vi "Host_17 - Copy - Copy.vi"() -> ()   [LabVIEW 2017]
uses:
  <vilib>/Platform/browser.llb/Open URL in Default Browser (string).vi
  <vilib>/lvdsc/tagapi/classes/Tag Reader/Tag Reader.lvclass
panel:
  in  "stop":bool
  out "Motor Speed":cluster{i32, dbl}[](graph)
  out "Armature Current":cluster{i32, dbl}[](graph)
  out "Feedback Load Torque 2":dbl
  out "Feedback Duty Cycle 2":dbl
  in  "Duty Cycle 2":dbl(slide) scale=0.0..100.0
  in  "Load Torque 2":dbl(slide) scale=-0.2..0.2
  in  "Data Update Speed (ms)":dbl
  in  "Website Button":bool
  in  "Doc Button":bool
  in  "Save Button":bool
  in  "Run Button":bool
  # "OPAL-RT Real Time Outputs"
  # "Microcontroller Inputs"
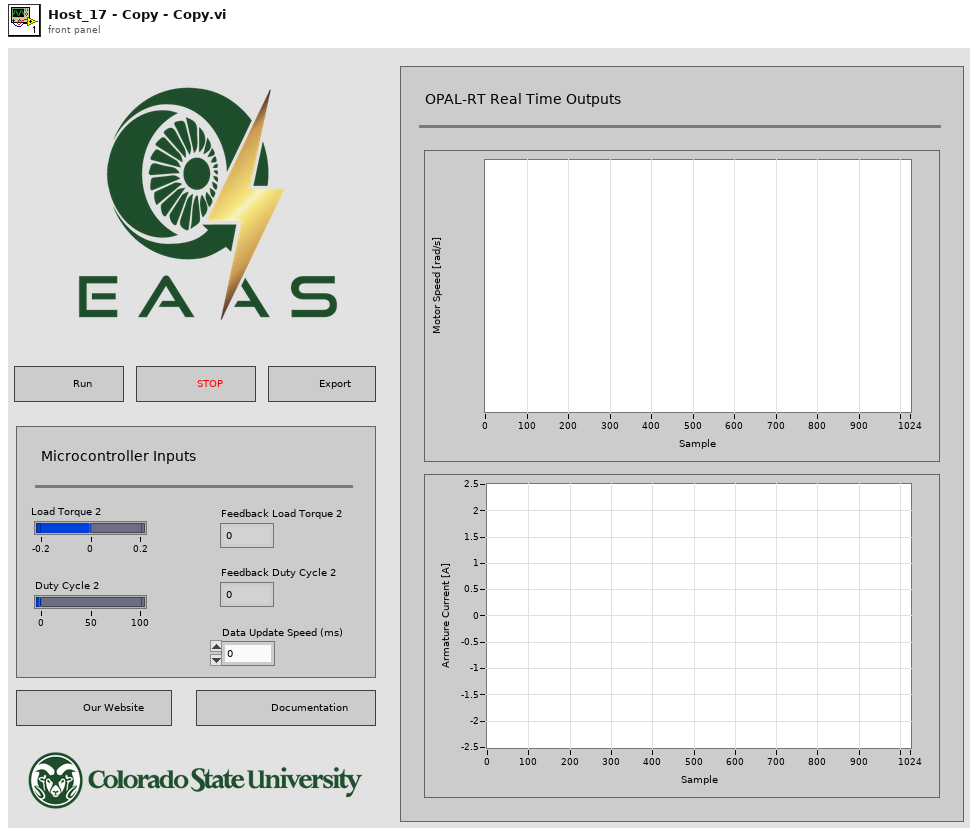
[diagram p1: front panel]
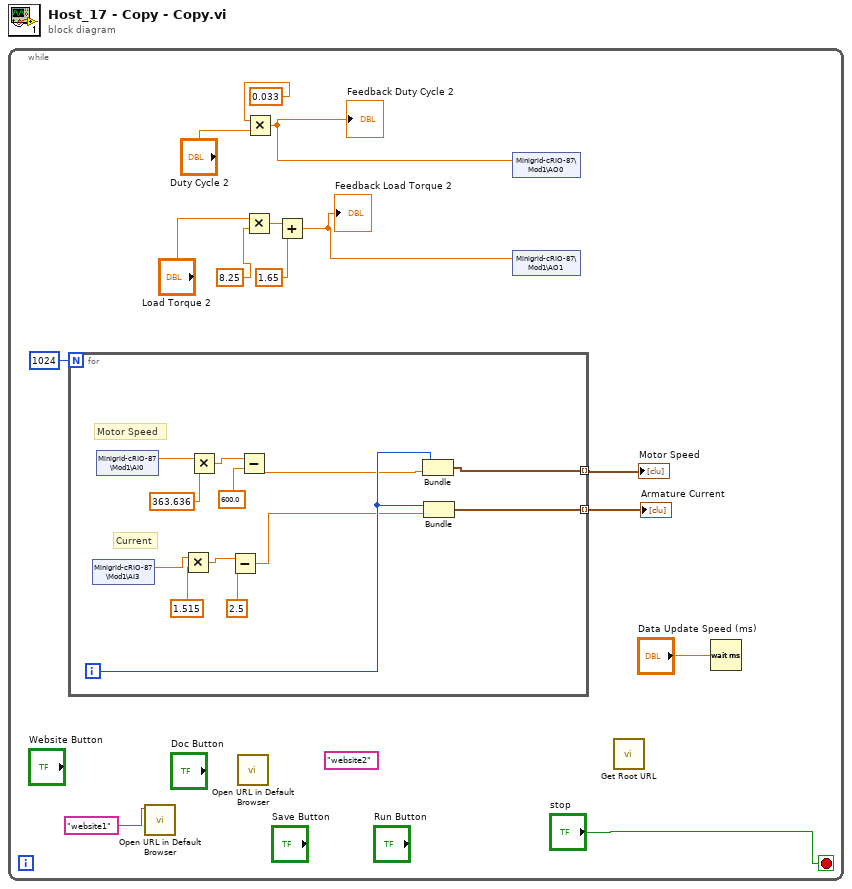
[diagram p0: block diagram]
diagram:
  n1 = while {
    stop <- "stop" stop-if-true
    (unwired) "website2"
    n2 = for {
      N: 1024 -> [_]
      tunnel: [w20] -> w13 mode=indexing
      tunnel: [w19] -> w2 mode=indexing
      i -> [w17]
      # "Current"
      # "Motor Speed"
      n3 = shared-variable "Minigrid-cRIO-87\\Mod1\\AI3"() -> (w18:dbl)  [unwired: 1 in, 1 out]
      n4 = shared-variable "Minigrid-cRIO-87\\Mod1\\AI0"() -> (w21:dbl)  [unwired: 1 in, 1 out]
      n5 = Multiply(x=w18, y=1.515) -> (x*y=w23:dbl)
      n6 = Multiply(x=w21, y=363.636) -> (x*y=w27:dbl)
      n7 = Subtract(x=w23, y=2.5) -> (x-y=w16:dbl)
      n8 = Subtract(x=w27, y=600.0) -> (x-y=w15:dbl)
      n9 = Bundle(w17, w15) -> (w19:cluster{i32, dbl})  [unwired: 1 in]
      n10 = Bundle(w17, w16) -> (w20:cluster{i32, dbl})  [unwired: 1 in]
    }
    "Armature Current" <- w13
    "Motor Speed" <- w2
    n11 = call-poly <vilib>:"Open URL in Default Browser.vi"("URL"="website1") -> ()  [unwired: 5 in, 2 out]
    n12 = call-poly <vilib>:"Open URL in Default Browser.vi"() -> ()  [unwired: 6 in, 2 out]
    n13 = Multiply(x="Load Torque 2", y=8.25) -> (x*y=w9:dbl)
    n14 = Multiply(x=0.033, y="Duty Cycle 2") -> (x*y=w6:dbl)
    "Feedback Duty Cycle 2" <- w6
    n15 = Add(x=w9, y=1.65) -> (x+y=w7:dbl)
    "Feedback Load Torque 2" <- w7
    n16 = shared-variable "Minigrid-cRIO-87\\Mod1\\AO0"(w6) -> ()  [unwired: 1 in, 1 out]
    n17 = shared-variable "Minigrid-cRIO-87\\Mod1\\AO1"(w7) -> ()  [unwired: 1 in, 1 out]
    n18 = call <vilib>:"Get Root URL.vi"() -> ()  [unwired: 9 in, 3 out]
    n19 = Wait (ms)(milliseconds to wait="Data Update Speed (ms)") -> ()  [unwired: 1 out]
  }
